vi "rwFile.vi"() -> ()   [LabVIEW 2016]
uses:
  <vilib>/Utility/file.llb/Write Delimited Spreadsheet (DBL).vi
  <vilib>/Utility/file.llb/Read Delimited Spreadsheet (DBL).vi
  <vilib>/regexp/Match Regular Expression.xnode
panel:
  in  "Clone?":bool
  in  "delimiter (\\t)":string=","
  in  "Z Array":dbl[](array[numeric])=[0.0, 0.0, 0.0, 0.0, 0.0, 0.0, 0.0, 0.0, 0.0, 0.0, 0.0, 0.0, 0.0, 0.0, 0.0, 0.0, 0.0, 0.0, 0.0, 0.0, 0.0, 0.0, 0.0, 0.0, 0.0, 0.0]
  in  "Y Array":dbl[](array[numeric])=[-32.0, -32.0, -32.0, -32.0, -32.0, -32.0, -32.0, -32.0, -32.0, -32.0, -32.0, -32.0, -32.0, -132.0, -132.0, -132.0, -132.0, -132.0, -132.0, -132.0, -132.0, -132.0, -132.0, -132.0, -132.0, -132.0]
  in  "X Array":dbl[](array[numeric])=[-709.0, -611.0, -513.0, -415.0, -317.0, -219.0, -121.0, -23.0, 75.0, 173.0, 271.0, 369.0, 467.0, 467.0, 369.0, 271.0, 173.0, 75.0, -23.0, -121.0, -219.0, -317.0, -415.0, -513.0, -611.0, -709.0]
  out "all rows":dbl[][](array[numeric])=[[-709.0, -32.0, 0.0], [-611.0, -32.0, 0.0], [-513.0, -32.0, 0.0], [-415.0, -32.0, 0.0], [-317.0, -32.0, 0.0], [-219.0, -32.0, 0.0], [-121.0, -32.0, 0.0], [-23.0, -32.0, 0.0], [75.0, -32.0, 0.0], [173.0, -32.0, 0.0], [271.0, -32.0, 0.0], [369.0, -32.0, 0.0], [467.0, -32.0, 0.0], [467.0, -132.0, 0.0], [369.0, -132.0, 0.0], [271.0, -132.0, 0.0], [173.0, -132.0, 0.0], [75.0, -132.0, 0.0], [-23.0, -132.0, 0.0], [-121.0, -132.0, 0.0], [-219.0, -132.0, 0.0], [-317.0, -132.0, 0.0], [-415.0, -132.0, 0.0], [-513.0, -132.0, 0.0], [-611.0, -132.0, 0.0], [-709.0, -132.0, 0.0]]
  in  "transpose? (no:F)":bool
  in  "file path (dialog if empty)":path=path "E:/XYZstage+Camera_CollectedImages/12-14-2016/nominalPOS_HighVoltageContacts.csv"
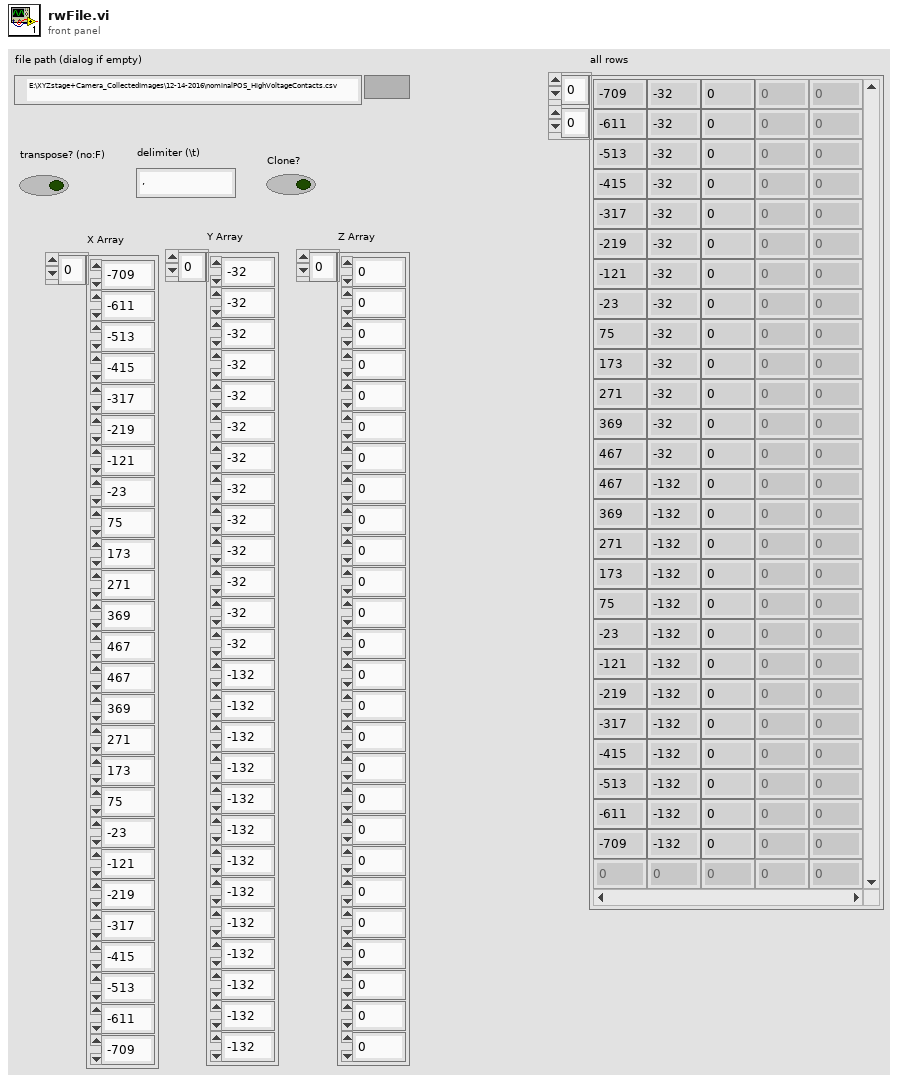
[diagram p1: front panel]
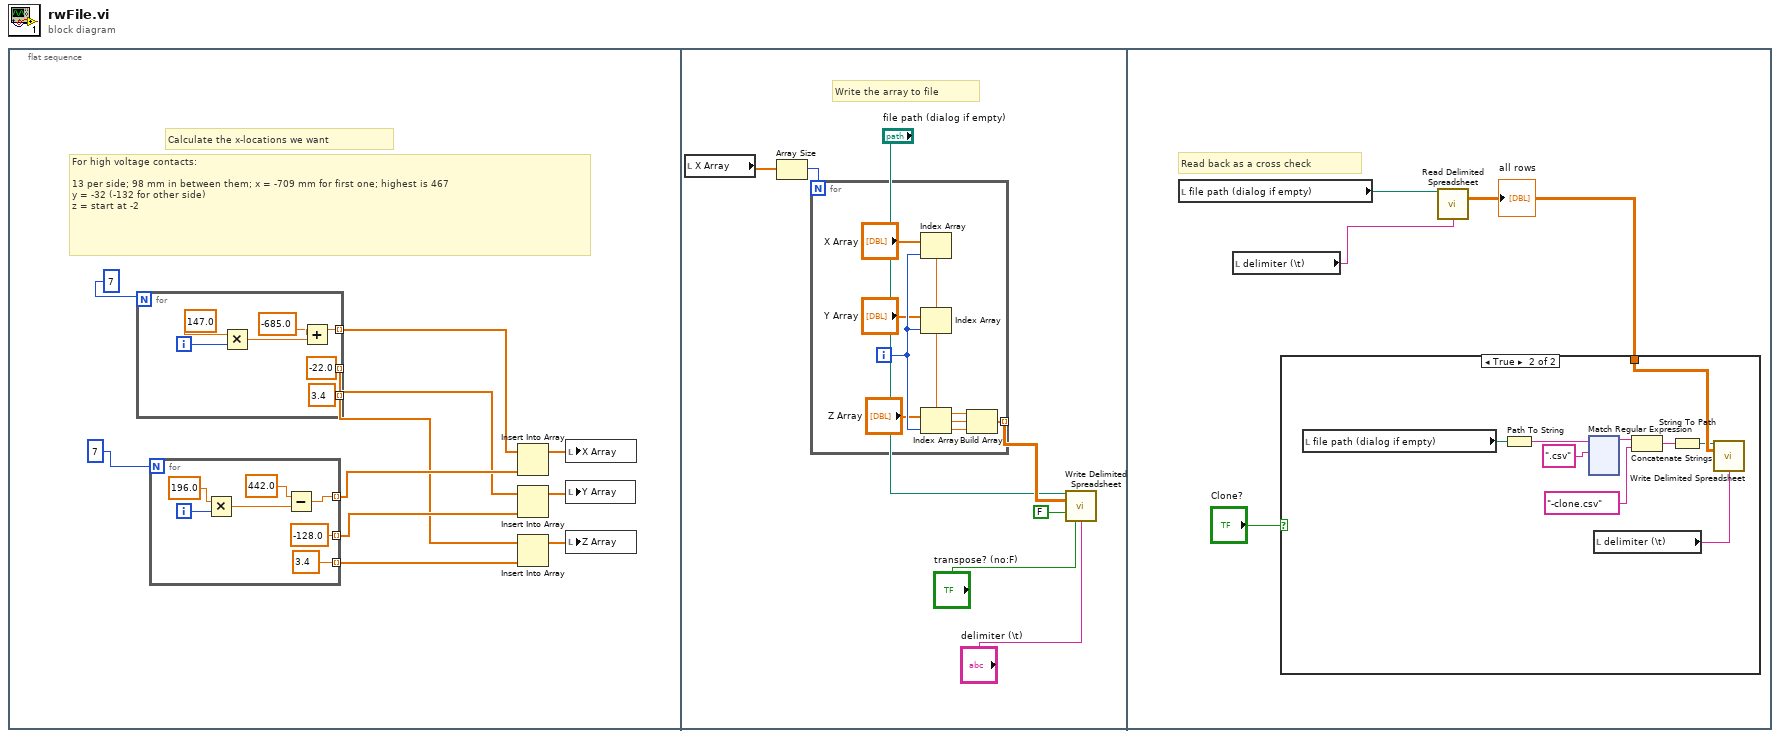
[diagram p0: block diagram]
diagram:
  n1 = flat-sequence {
    frame #0 {
      # "For high voltage contacts:\n\n13 per side; 98 mm in between them; x = -709 mm for first one; highest is 467 \ny = -32 (-132 for other side) \nz = start at -2"
      # "Calculate the x-locations we want"
      n2 = for {
        N: 7 -> [_]
        tunnel: [-22.0] -> w6 mode=indexing
        tunnel: [w16] -> w9 mode=indexing
        tunnel: [3.4] -> w4 mode=indexing
        i -> [w15]
        n3 = Multiply(x=147.0, y=w15) -> (x*y=w12:dbl)
        n4 = Add(x=-685.0, y=w12) -> (x+y=w16:dbl)
      }
      n5 = for {
        N: 7 -> [_]
        tunnel: [-128.0] -> w5 mode=indexing
        tunnel: [w23] -> w8 mode=indexing
        tunnel: [3.4] -> w3 mode=indexing
        i -> [w22]
        n6 = Multiply(x=196.0, y=w22) -> (x*y=w19:dbl)
        n7 = Subtract(x=442.0, y=w19) -> (x-y=w23:dbl)
      }
      n8 = Insert Into Array(array=w9, new element=w8) -> (w7:dbl[])  [unwired: 1 in]
      n9 = Insert Into Array(array=w6, new element=w5) -> (w1:dbl[])  [unwired: 1 in]
      n10 = Insert Into Array(array=w4, new element=w3) -> (w2:dbl[])  [unwired: 1 in]
      n11 = local write "X Array"(w7) -> ()
      n12 = local write "Y Array"(w1) -> ()
      n13 = local write "Z Array"(w2) -> ()
    }
    frame #1 {
      # "Write the array to file"
      n14 = local read "X Array"() -> (w30:dbl[])
      n15 = Array Size(array=w30) -> (size(s)=w29:i32)
      n16 = for {
        N: w29 -> [_]
        tunnel: [w33] -> w31 mode=indexing
        i -> [w40]
        n17 = Index Array(array="X Array", index=w40) -> (element=w34:dbl)
        n18 = Index Array(array="Y Array", index=w40) -> (element=w36:dbl)
        n19 = Index Array(array="Z Array", index=w40) -> (element=w35:dbl)
        n20 = Build Array(w34, w36, w35) -> (w33:dbl[])
      }
      n21 = call-poly <vilib>:"Write Delimited Spreadsheet.vi"("file path (dialog if empty)"="file path (dialog if empty)", "2D data"=w31, "append to file? (new file:F)"=FALSE, "transpose? (no:F)"="transpose? (no:F)", "delimiter (\\t)"="delimiter (\\t)") -> ()  [unwired: 9 in, 2 out]
    }
    frame #2 {
      # "Read back as a cross check"
      n22 = local read "file path (dialog if empty)"() -> (w44:path)
      n23 = local read "delimiter (\\t)"() -> (w41:string)
      n24 = call-poly <vilib>:"Read Delimited Spreadsheet.vi"("file path (dialog if empty)"=w44, "delimiter (\\t)"=w41) -> ("all rows"=w43:dbl[][])  [unwired: 8 in, 5 out]
      "all rows" <- w43
      n25 = case shown="True" "Clone?" {
        tunnel: w43 -> [_ w53]
        frame False {
        }
        frame True {
          n26 = local read "file path (dialog if empty)"() -> (w52:path)
          n27 = Path To String(path=w52) -> (string=w51:string)
          n28 = xnode "Match Regular Expression"("input string"=w51, "regular expression"=".csv") -> ("before match"=w48:string)  [unwired: 4 in, 4 out]
          n29 = local read "delimiter (\\t)"() -> (w45:string)
          n30 = Concatenate Strings(w48, "-clone.csv" ("name or relative path")) -> (w47:string)
          n31 = String To Path(string=w47) -> (path=w46:path)
          n32 = call-poly <vilib>:"Write Delimited Spreadsheet.vi"("file path (dialog if empty)"=w46, "2D data"=w53, "delimiter (\\t)"=w45) -> ()  [unwired: 11 in, 2 out]
        }
      }
    }
  }
